vi "sub UI get basic data.vi"(8 "error in (no error)":errorcluster, 11 "IDE simple in":refnum<class "LF2R IDE.lvclass">) -> (0 "error out":errorcluster, 2 "frame basic data":T1, 3 "IDE simple out":refnum<class "LF2R IDE.lvclass">)   [LabVIEW 2018, in "LF2R IDE.lvlib" / "LF2R IDE.lvclass"]
uses:
  LF2R IDE.lvclass
  Frame Analizer/frame basic data.ctl
  LF2R IDE.lvclass/LF2R IDE.ctl
  Frame Analizer/Data Parser.lvclass
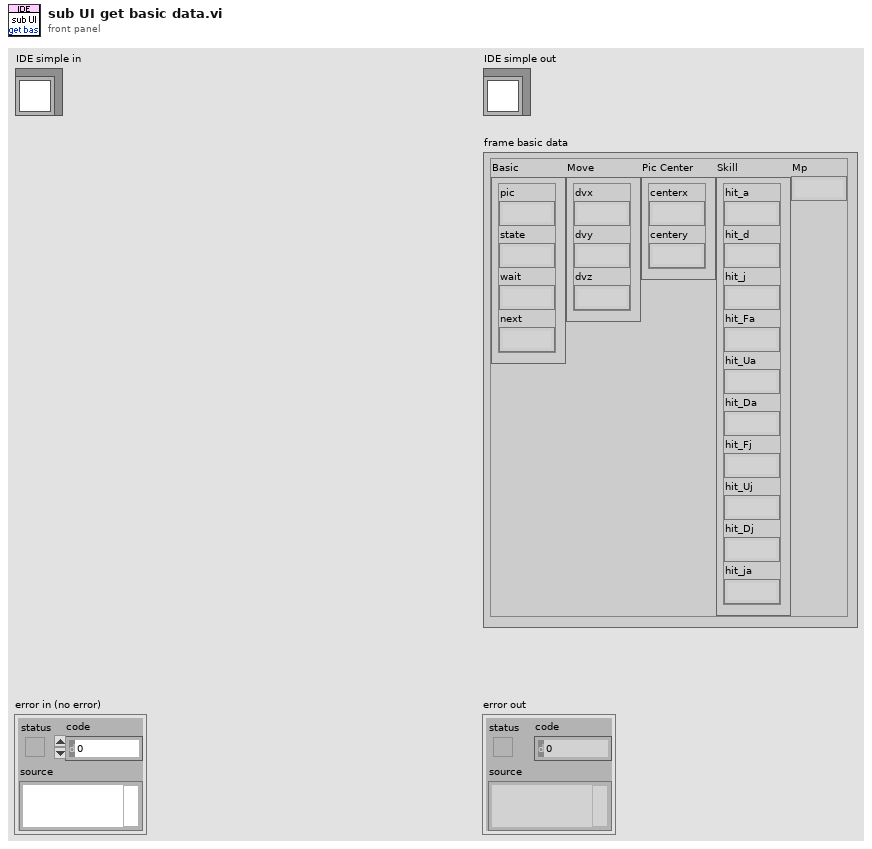
[diagram p1: front panel]
types:
  T1 = typedef "Data Parser.lvclass/frame basic data.ctl" = cluster{"Basic":cluster{"pic":string, "state":string, "wait":string, "next":string}, "Move":cluster{"dvx":string, "dvy":string, "dvz":string}, "Pic Center":cluster{"centerx":string, "centery":string}, "Skill":cluster{"hit_a":string, "hit_d":string, "hit_j":string, "hit_Fa":string, "hit_Ua":string, "hit_Da":string, "hit_Fj":string, "hit_Uj":string, "hit_Dj":string, "hit_ja":string}, "Mp":string}
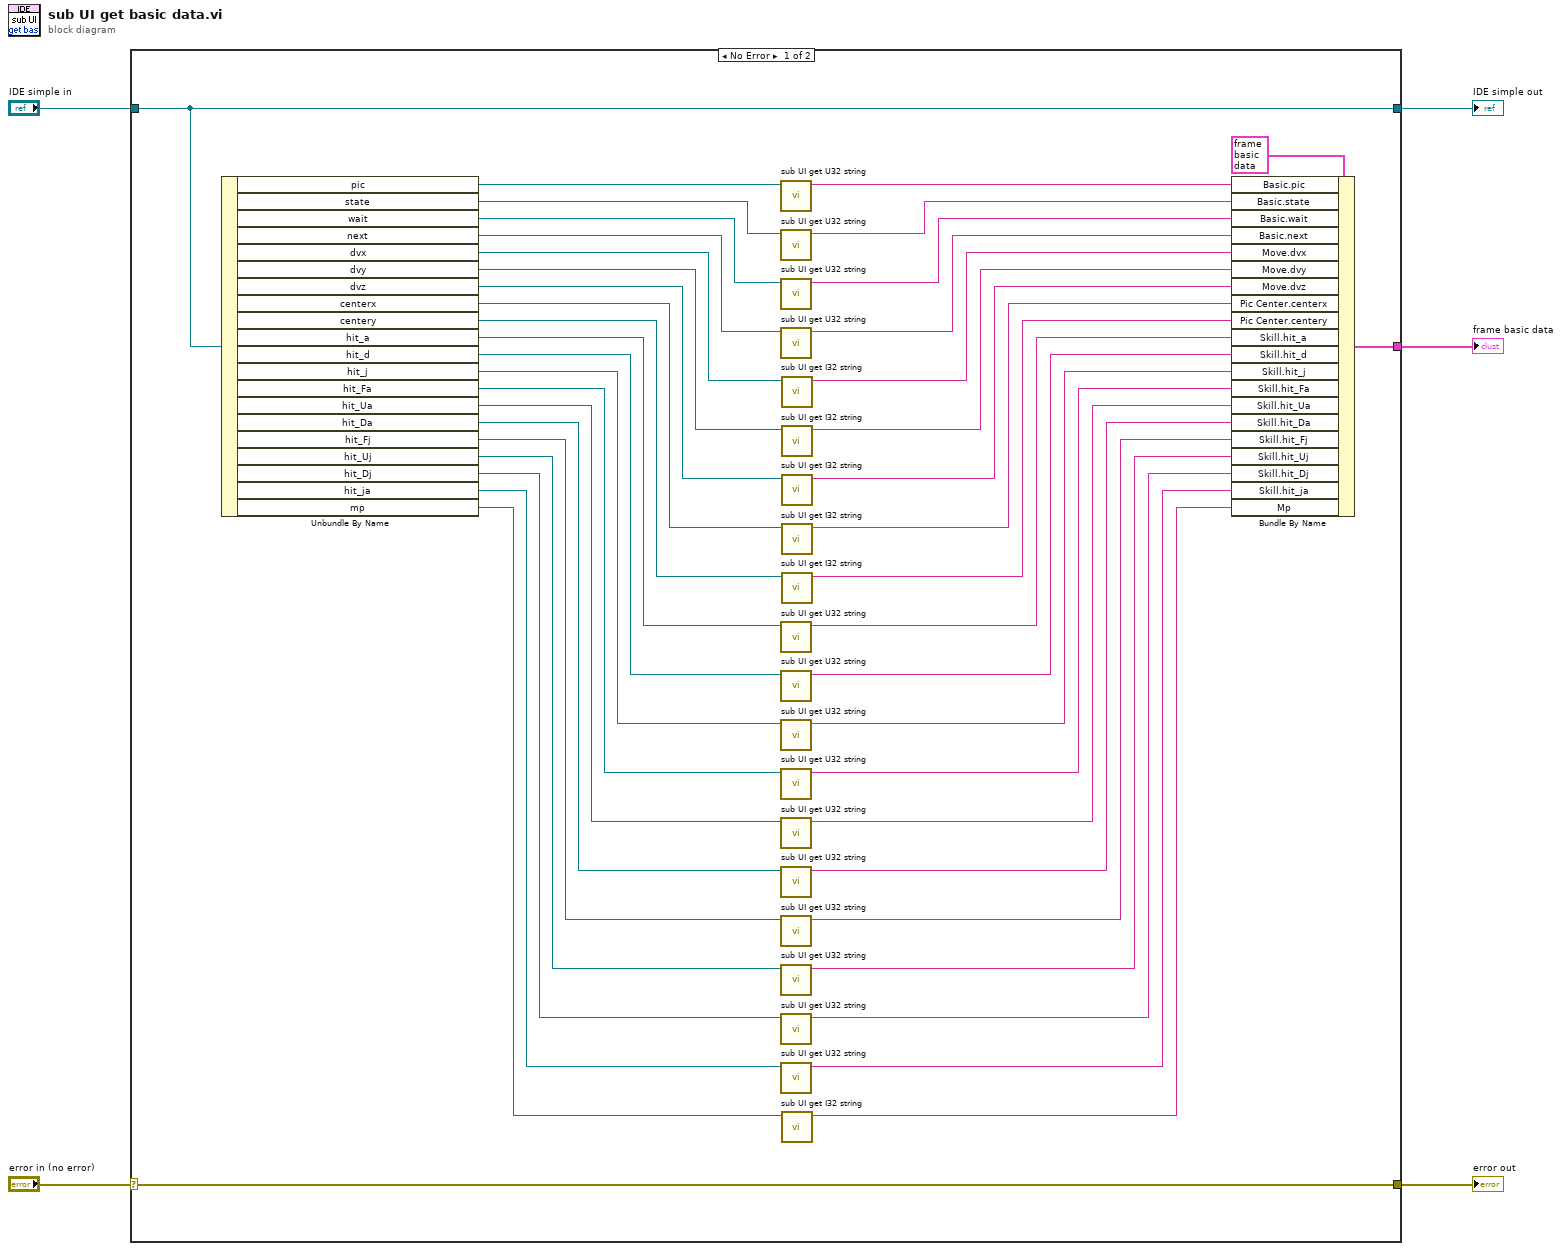
[diagram p0: block diagram]
diagram:
  n1 = case shown="No Error" "error in (no error)" {
    selector: "error in (no error)" -> [w6 w51]
    tunnel: [w6 w51] -> w4
    tunnel: [w49 w50] -> w2
    tunnel: "IDE simple in" -> [w49 w50]
    tunnel: [w48 _] -> w1
    frame No Error {
      n2 = Unbundle By Name(w49) -> ("pic"=w46:refnum<vi>, "state"=w45:refnum<vi>, "wait"=w44:refnum<vi>, "next"=w43:refnum<vi>, "dvx"=w42:refnum<vi>, "dvy"=w41:refnum<vi>, "dvz"=w40:refnum<vi>, "centerx"=w39:refnum<vi>, "centery"=w38:refnum<vi>, "hit_a"=w37:refnum<vi>, "hit_d"=w36:refnum<vi>, "hit_j"=w35:refnum<vi>, "hit_Fa"=w34:refnum<vi>, "hit_Ua"=w33:refnum<vi>, "hit_Da"=w32:refnum<vi>, "hit_Fj"=w31:refnum<vi>, "hit_Uj"=w30:refnum<vi>, "hit_Dj"=w29:refnum<vi>, "hit_ja"=w28:refnum<vi>, "mp"=w27:refnum<vi>)
      n3 = call "sub UI get U32 string.vi"("U32 Ref"=w46) -> ("Value string"=w26:string)  [unwired: 9 in, 1 out]
      n4 = call "sub UI get U32 string.vi"("U32 Ref"=w45) -> ("Value string"=w25:string)  [unwired: 9 in, 1 out]
      n5 = call "sub UI get U32 string.vi"("U32 Ref"=w44) -> ("Value string"=w24:string)  [unwired: 9 in, 1 out]
      n6 = call "sub UI get U32 string.vi"("U32 Ref"=w43) -> ("Value string"=w23:string)  [unwired: 9 in, 1 out]
      n7 = call "sub UI get U32 string.vi"("U32 Ref"=w37) -> ("Value string"=w17:string)  [unwired: 9 in, 1 out]
      n8 = call "sub UI get U32 string.vi"("U32 Ref"=w36) -> ("Value string"=w16:string)  [unwired: 9 in, 1 out]
      n9 = call "sub UI get U32 string.vi"("U32 Ref"=w35) -> ("Value string"=w15:string)  [unwired: 9 in, 1 out]
      n10 = call "sub UI get U32 string.vi"("U32 Ref"=w34) -> ("Value string"=w14:string)  [unwired: 9 in, 1 out]
      n11 = call "sub UI get U32 string.vi"("U32 Ref"=w33) -> ("Value string"=w13:string)  [unwired: 9 in, 1 out]
      n12 = call "sub UI get U32 string.vi"("U32 Ref"=w32) -> ("Value string"=w12:string)  [unwired: 9 in, 1 out]
      n13 = call "sub UI get U32 string.vi"("U32 Ref"=w31) -> ("Value string"=w11:string)  [unwired: 9 in, 1 out]
      n14 = call "sub UI get U32 string.vi"("U32 Ref"=w30) -> ("Value string"=w10:string)  [unwired: 9 in, 1 out]
      n15 = call "sub UI get U32 string.vi"("U32 Ref"=w29) -> ("Value string"=w9:string)  [unwired: 9 in, 1 out]
      n16 = call "sub UI get U32 string.vi"("U32 Ref"=w28) -> ("Value string"=w8:string)  [unwired: 9 in, 1 out]
      n17 = call "sub UI get I32 string.vi"("I32 Ref"=w42) -> ("Value string"=w22:string)  [unwired: 9 in, 1 out]
      n18 = call "sub UI get I32 string.vi"("I32 Ref"=w41) -> ("Value string"=w21:string)  [unwired: 9 in, 1 out]
      n19 = call "sub UI get I32 string.vi"("I32 Ref"=w40) -> ("Value string"=w20:string)  [unwired: 9 in, 1 out]
      n20 = call "sub UI get I32 string.vi"("I32 Ref"=w39) -> ("Value string"=w19:string)  [unwired: 9 in, 1 out]
      n21 = call "sub UI get I32 string.vi"("I32 Ref"=w38) -> ("Value string"=w18:string)  [unwired: 9 in, 1 out]
      n22 = call "sub UI get I32 string.vi"("I32 Ref"=w27) -> ("Value string"=w7:string)  [unwired: 9 in, 1 out]
      n23 = Bundle By Name(cluster=T1 {"Basic"={"pic"="", "state"="", "wait"="", "next"=""}, "Move"={"dvx"="", "dvy"="", "dvz"=""}, "Pic Center"={"centerx"="", "centery"=""}, "Skill"={"hit_a"="", "hit_d"="", "hit_j"="", "hit_Fa"="", "hit_Ua"="", "hit_Da"="", "hit_Fj"="", "hit_Uj"="", "hit_Dj"="", "hit_ja"=""}, "Mp"=""} ("frame basic data"), "Basic.pic"=w26, "Basic.state"=w25, "Basic.wait"=w24, "Basic.next"=w23, "Move.dvx"=w22, "Move.dvy"=w21, "Move.dvz"=w20, "Pic Center.centerx"=w19, "Pic Center.centery"=w18, "Skill.hit_a"=w17, "Skill.hit_d"=w16, "Skill.hit_j"=w15, "Skill.hit_Fa"=w14, "Skill.hit_Ua"=w13, "Skill.hit_Da"=w12, "Skill.hit_Fj"=w11, "Skill.hit_Uj"=w10, "Skill.hit_Dj"=w9, "Skill.hit_ja"=w8, "Mp"=w7) -> (w48:T1)
    }
    frame Error {
    }
  }
  "error out" <- w4
  "IDE simple out" <- w2
  "frame basic data" <- w1
